vi "m1m3_getEvent_DisplacementSensorWarning.vi"(8 "error in (no error)":errorcluster, 11 "logevent_DisplacementSensorWarning_Ctl":T1) -> (0 "error out":errorcluster, 2 "function return":i32, 3 "logevent_DisplacementSensorWarning_Ctl out":T1)   [LabVIEW 2016, in "SALLV_m1m3.lvlib"]
doc: "int m1m3_shm_getEvent_DisplacementSensorWarningLV(m1m3_logevent_DisplacementSensorWarningLV *logevent_DisplacementSensorWarning_Ctl );"
uses:
  SALLV_m1m3.lvlib
  DataTypes/logevent_DisplacementSensorWarning.ctl
  SALLV_m1m3.so
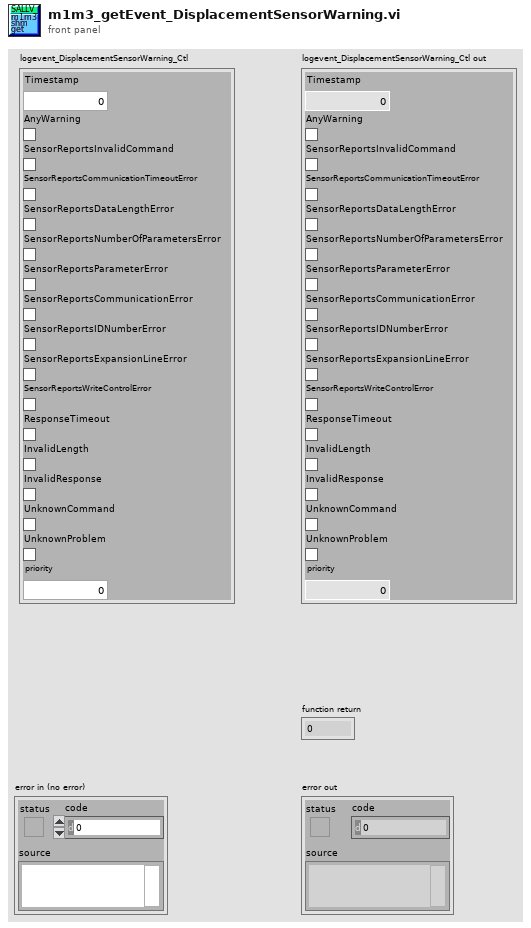
[diagram p1: front panel]
types:
  T1 = typedef "SALLV_m1m3.lvlib/logevent_DisplacementSensorWarning.ctl" = cluster{"Timestamp":dbl, "AnyWarning":bool, "SensorReportsInvalidCommand":bool, "SensorReportsCommunicationTimeoutError":bool, "SensorReportsDataLengthError":bool, "SensorReportsNumberOfParametersError":bool, "SensorReportsParameterError":bool, "SensorReportsCommunicationError":bool, "SensorReportsIDNumberError":bool, "SensorReportsExpansionLineError":bool, "SensorReportsWriteControlError":bool, "ResponseTimeout":bool, "InvalidLength":bool, "InvalidResponse":bool, "UnknownCommand":bool, "UnknownProblem":bool, "priority":i32}
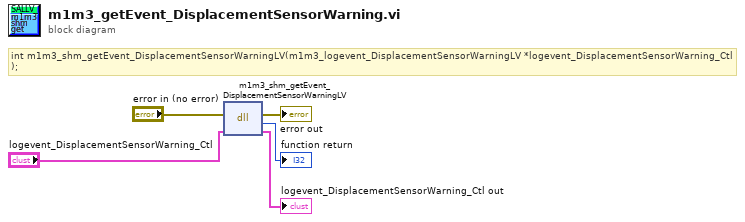
[diagram p0: block diagram]
diagram:
  # "int m1m3_shm_getEvent_DisplacementSensorWarningLV(m1m3_logevent_DisplacementSensorWarningLV *logevent_DisplacementSensorWarning_Ctl );"
  n1 = dll-call lib="opt/CODE/SALLV_m1m3/SALLV_m1m3.*" fn="m1m3_shm_getEvent_DisplacementSensorWarningLV"(error in="error in (no error)", "logevent_DisplacementSensorWarning_Ctl"="logevent_DisplacementSensorWarning_Ctl") -> (error out=→"error out":errorcluster, →"function return":i32, "logevent_DisplacementSensorWarning_Ctl"=→"logevent_DisplacementSensorWarning_Ctl out":T1)  [unwired: 2 in, 1 out]
